vi "StreamTransmitTCS-RS232.vi"() -> ()   [LabVIEW 2018]
uses:
  <vilib>/Instr/_visa.llb/VISA Configure Serial Port (Instr).vi
panel:
  out "VISA resource name out":refnum<visa-resource-name>
  in  "Input Cluster":T1={"baud rate (9600)"=2400, "VISA resource name"=""}
  out "error out 2":errorcluster
  in  "stop":bool
  out "error out":errorcluster
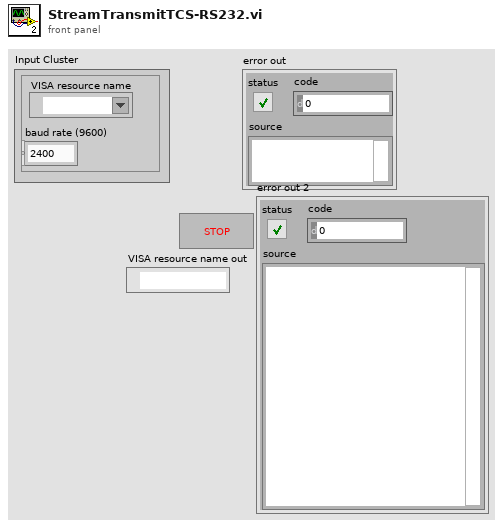
[diagram p1: front panel]
types:
  T1 = cluster{"baud rate (9600)":u32, "VISA resource name":refnum<visa-resource-name>}
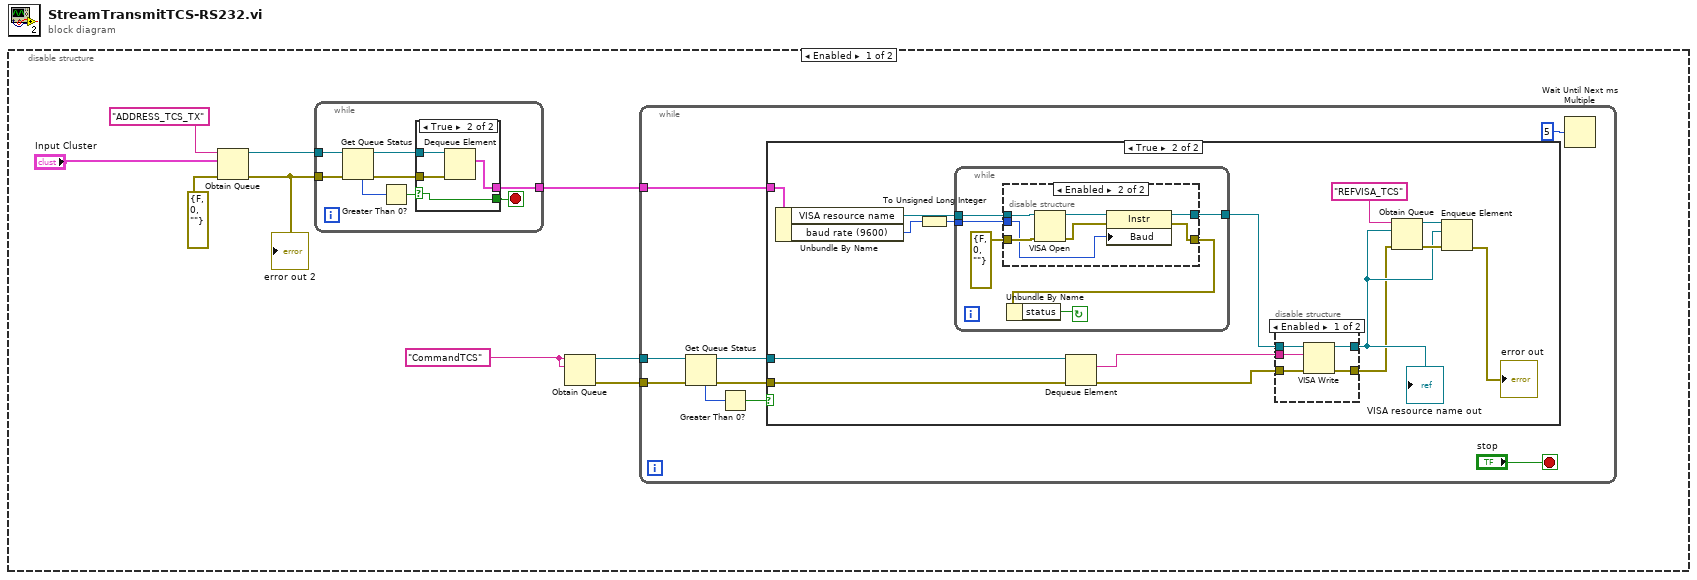
[diagram p0: block diagram]
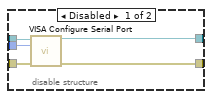
[diagram p5: hidden frame]
diagram:
  n1 = disable-structure shown="Enabled" {
    frame Enabled {
      w8 = "CommandTCS"
      n2 = Obtain Queue(name (unnamed)="ADDRESS_TCS_TX", element data type="Input Cluster", error in (no error)=errorcluster {"status"=FALSE, "code"=0, "source"=""}) -> (queue out=w5:refnum<queue>, error out=w6:errorcluster)  [unwired: 2 in, 1 out]
      "error out 2" <- w6
      n3 = while {
        tunnel: [w17] -> w4
        tunnel: w6 -> [w15]
        tunnel: w5 -> [w14]
        stop <- w10 stop-if-true
        n4 = Get Queue Status(queue=w14, error in (no error)=w15) -> (queue out=w13:refnum<queue>, error out=w16:errorcluster, # elements in queue=w12:i32)  [unwired: 1 in, 5 out]
        n5 = Greater Than 0?(x=w12) -> (x > 0?=w11:bool)
        n6 = case shown="True" w11 {
          selector: w11 -> [w18 w19]
          tunnel: [_ w22] -> w17
          tunnel: w16 -> [_ w21]
          tunnel: w13 -> [_ w20]
          tunnel: [w18 w19] -> w10
          frame False {
          }
          frame True {
            n7 = Dequeue Element(queue=w20, error in (no error)=w21) -> (element=w22:T1)  [unwired: 1 in, 3 out]
          }
        }
      }
      n8 = Obtain Queue(name (unnamed)=w8, element data type=w8) -> (queue out=w9:refnum<queue>, error out=w3:errorcluster)  [unwired: 3 in, 1 out]
      n9 = while {
        tunnel: w9 -> [w30]
        tunnel: w4 -> [w23]
        tunnel: w3 -> [w25]
        stop <- "stop" stop-if-true
        n10 = Get Queue Status(queue=w30, error in (no error)=w25) -> (queue out=w27:refnum<queue>, error out=w24:errorcluster, # elements in queue=w29:i32)  [unwired: 1 in, 5 out]
        n11 = Greater Than 0?(x=w29) -> (x > 0?=w28:bool)
        n12 = case shown="True" w28 {
          tunnel: w27 -> [_ w46]
          tunnel: w24 -> [_ w38]
          tunnel: w23 -> [_ w32]
          frame False {
          }
          frame True {
            n13 = Unbundle By Name(w32) -> ("VISA resource name"=w35:refnum<visa-resource-name>, "baud rate (9600)"=w36:u32)
            n14 = To Unsigned Long Integer(number=w36) -> (unsigned 32bit integer=w34:u32)
            n15 = while {
              tunnel: w34 -> [w57]
              tunnel: w35 -> [w58]
              tunnel: [w54] -> w33
              stop <- w59 continue-if-true
              n16 = disable-structure shown="Enabled" {
                disable-tunnel: w58 -> [w64 w71]
                disable-tunnel: w57 -> [w63 w65]
                disable-tunnel: errorcluster {"status"=FALSE, "code"=0, "source"=""} ("error in (no error)") -> [w62 w70]
                disable-tunnel: [w61 w66] -> w55
                disable-tunnel: [w60 w68] -> w54
                frame Disabled {
                  n17 = call-poly "VISA Configure Serial Port"("VISA resource name"=w64, "baud rate (9600)"=w63, "error in (no error)"=w62) -> ("VISA resource name out"=w60:refnum<visa-resource-name>, "error out"=w61:errorcluster)  [unwired: 11 in]
                }
                frame Enabled {
                  n18 = VISA Open(error in (no error)=w70, VISA resource name=w71) -> (VISA resource name=w69:refnum<visa-resource-name>, error out=w67:errorcluster)  [unwired: 3 in]
                  n19 = property class="Instr"(reference=w69, error in=w67, "Baud"=w65) -> (reference out=w68:refnum<visa-resource-name>, error out=w66:errorcluster)
                }
              }
              n20 = Unbundle By Name(w55) -> ("status"=w59:bool)
            }
            n21 = Dequeue Element(queue=w46, error in (no error)=w38) -> (element=w41:string, error out=w37:errorcluster)  [unwired: 1 in, 2 out]
            n22 = disable-structure shown="Enabled" {
              disable-tunnel: w41 -> [w51 _]
              disable-tunnel: [w50 w53] -> w40
              disable-tunnel: [w49 w52] -> w39
              disable-tunnel: w37 -> [w48 w52]
              disable-tunnel: w33 -> [w47 w53]
              frame Enabled {
                n23 = VISA Write(VISA resource name=w47, write buffer=w51, error in (no error)=w48) -> (VISA resource name out=w50:refnum<visa-resource-name>, error out=w49:errorcluster)  [unwired: 1 out]
              }
              frame Disabled {
              }
            }
            "VISA resource name out" <- w40
            n24 = Obtain Queue(name (unnamed)="REFVISA_TCS", element data type=w40, error in (no error)=w39) -> (queue out=w43:refnum<queue>, error out=w44:errorcluster)  [unwired: 2 in, 1 out]
            n25 = Enqueue Element(queue=w43, element=w40, error in (no error)=w44) -> (error out=→"error out":errorcluster)  [unwired: 1 in, 2 out]
          }
        }
        n26 = Wait Until Next ms Multiple(millisecond multiple=u32 5) -> ()  [unwired: 1 out]
      }
    }
    frame Disabled {
    }
  }
